vi "HomeStage.vi"(8 "error in":errorcluster, 9 "Stage":T1, 11 "reference in":refnum<k7>) -> (0 "error out":errorcluster, 2 "result string":string, 3 "reference out":refnum<k7>)   [LabVIEW 2020]
uses:
  StageSelector--Enum.ctl
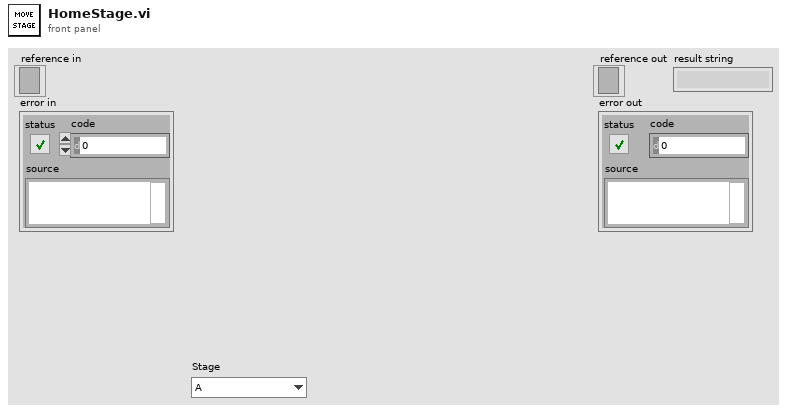
[diagram p1: front panel]
types:
  T1 = typedef "StageSelector--Enum.ctl" = enum16{"A", "B", "C", "D"}
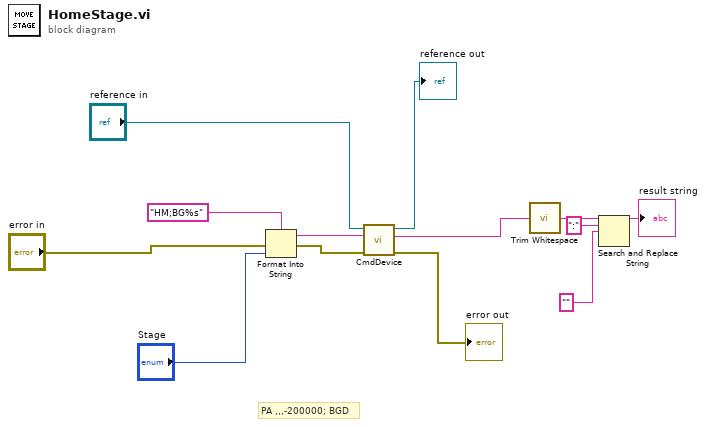
[diagram p0: block diagram]
diagram:
  # "PA ,,,-200000; BGD"
  n1 = Format Into String(format string="HM;BG%s", error in="error in", "Stage") -> (resulting string=w1:string, error out=w10:errorcluster)  [unwired: 1 in]
  n2 = call "CmdDevice.vi"("error in (no error)"=w10, "Command:"=w1, "reference in"="reference in") -> ("error out"=→"error out":errorcluster, "Response:"=w3:string, "reference out"=→"reference out":refnum<k7>)  [unwired: 6 in]
  n3 = call <vilib>:"Trim Whitespace.vi"("string"=w3) -> ("trimmed string"=w6:string)  [unwired: 1 in]
  n4 = Search and Replace String(input string=w6, search string=":", replace string="" ("replace string (\"\")")) -> (result string=→"result string":string)  [unwired: 5 in, 3 out]
